vi "Load Application Config.vi"(8 "error in":errorcluster, 10 "Config path":path=path "C:/GitHub/OOP_Submodule EOL/Config/INI Config.ini", 11 "Sequence Context In":refnum<k7>) -> (0 "error out":errorcluster)   [LabVIEW 2021]
uses:
  <vilib>/Utility/config.llb/Read Key (String).vi
  <vilib>/addons/TestStand/_TSUtility.llb/TestStand - Set Property Value (String).vi
  <vilib>/addons/TestStand/_TSUtility.llb/TestStand - Set Property Value (Number).vi
  <vilib>/Utility/config.llb/NI_LVConfig.lvlib
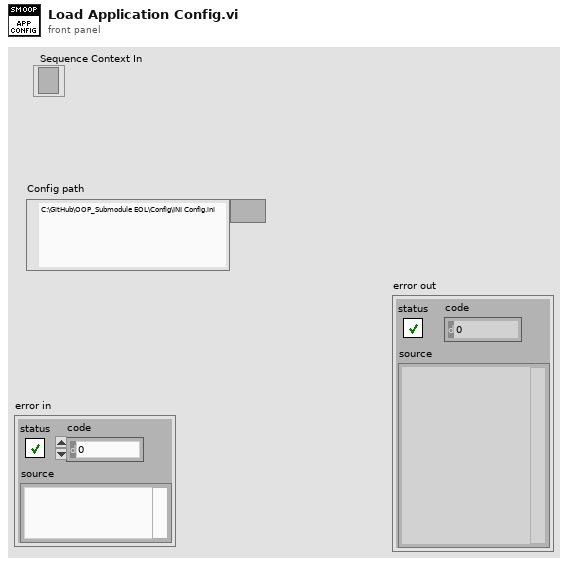
[diagram p1: front panel]
types:
  T1 = typedef "NI_LVConfig.lvlib/Config Data RefNum.ctl" = refnum<k1>
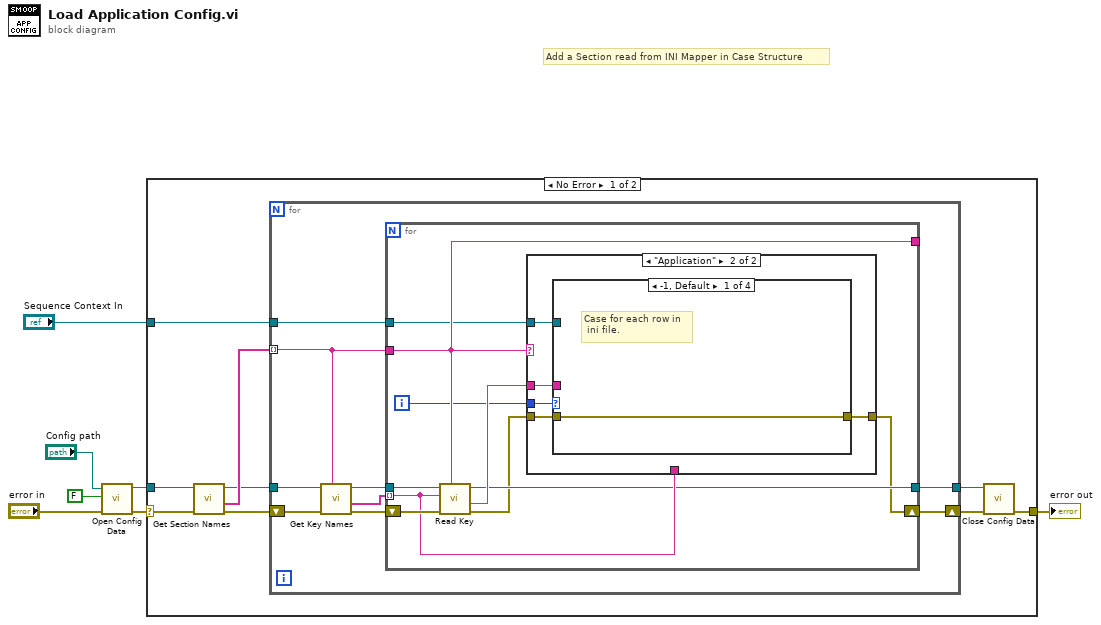
[diagram p0: block diagram]
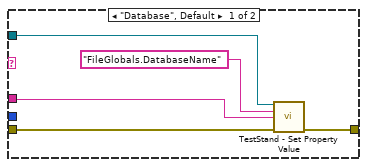
[diagram p2: hidden frame]
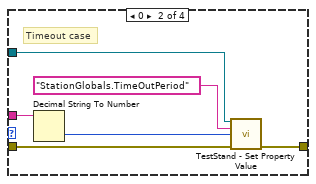
[diagram p3: hidden frame]
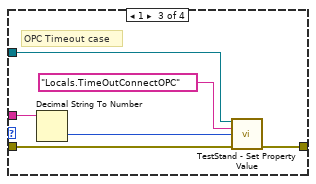
[diagram p4: hidden frame]
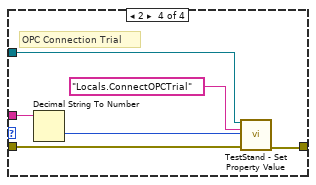
[diagram p5: hidden frame]
diagram:
  # "Add a Section read from INI Mapper in Case Structure"
  n1 = call <vilib>:"Open Config Data.vi"("error in (no error)"="error in", "create file if necessary (T)"=FALSE, "configuration file path"="Config path") -> ("error out"=w5:errorcluster, "refnum"=w6:T1)  [unwired: 6 in, 1 out]
  n2 = case shown="No Error" w5 {
    selector: w5 -> [w16 w65]
    tunnel: [w9 w65] -> w2
    tunnel: w6 -> [w15 _]
    tunnel: "Sequence Context In" -> [w8 _]
    frame No Error {
      n3 = call <vilib>:"Get Section Names.vi"("error in (no error)"=w16, "refnum"=w15) -> ("error out"=w13:errorcluster, "section names"=w14:string[], "refnum out"=w12:T1)  [unwired: 7 in]
      n4 = for {
        tunnel: w14 -> [w22] mode=indexing
        tunnel: w12 -> [w24]
        tunnel: [w23] -> w11
        shift-right: [w18] -> w10
        shift-left: w13 -> [w25]
        tunnel: w8 -> [w17]
        n5 = call <vilib>:"Get Key Names.vi"("section"=w22, "error in (no error)"=w25, "refnum"=w24) -> ("error out"=w21:errorcluster, "key names"=w20:string[], "refnum out"=w19:T1)  [unwired: 5 in, 1 out]
        n6 = for {
          tunnel: w20 -> [w33] mode=indexing
          tunnel: w22 -> [w30]
          tunnel: w19 -> [w34]
          tunnel: [w31] -> w23
          tunnel: [w30] -> _
          shift-right: [w26] -> w18
          shift-left: w21 -> [w35]
          tunnel: w17 -> [w29]
          i -> [w28]
          n7 = call-poly <vilib>:"Read Key.vi"("section"=w30, "error in (no error)"=w35, "key"=w33, "refnum"=w34) -> ("error out"=w27:errorcluster, "value"=w32:string, "refnum out"=w31:T1)  [unwired: 4 in, 1 out]
          n8 = case shown="\"Application\"" w30 {
            tunnel: w33 -> [_ _]
            tunnel: w32 -> [w39 w45]
            tunnel: w29 -> [w38 w43]
            tunnel: w28 -> [_ w44]
            tunnel: w27 -> [w37 w42]
            tunnel: [w36 w41] -> w26
            frame "Database", Default {
              n9 = call-poly <vilib>:"TestStand - Set Property Value.vi"("Sequence Context In"=w38, "Lookup String"="FileGlobals.DatabaseName", "New Value"=w39, "error in (no error)"=w37) -> ("error out"=w36:errorcluster)  [unwired: 10 in, 1 out]
            }
            frame "Application" {
              n10 = case shown="-1, Default" w44 {
                tunnel: w45 -> [_ w51 w57 w63]
                tunnel: w43 -> [_ w49 w55 w61]
                tunnel: w42 -> [w46 w48 w54 w60]
                tunnel: [w46 w47 w53 w59] -> w41
                frame -1, Default {
                  # "Case for each row in\n ini file."
                }
                frame 0 {
                  # "Timeout case"
                  n11 = Decimal String To Number(string=w51) -> (number=w50:i32)  [unwired: 2 in, 1 out]
                  n12 = call-poly <vilib>:"TestStand - Set Property Value.vi"("Sequence Context In"=w49, "Lookup String"="StationGlobals.TimeOutPeriod", "New Value"=w50, "error in (no error)"=w48) -> ("error out"=w47:errorcluster)  [unwired: 10 in, 1 out]
                }
                frame 1 {
                  # "OPC Timeout case"
                  n13 = Decimal String To Number(string=w57) -> (number=w56:i32)  [unwired: 2 in, 1 out]
                  n14 = call-poly <vilib>:"TestStand - Set Property Value.vi"("Sequence Context In"=w55, "Lookup String"="Locals.TimeOutConnectOPC", "New Value"=w56, "error in (no error)"=w54) -> ("error out"=w53:errorcluster)  [unwired: 10 in, 1 out]
                }
                frame 2 {
                  # "OPC Connection Trial"
                  n15 = Decimal String To Number(string=w63) -> (number=w62:i32)  [unwired: 2 in, 1 out]
                  n16 = call-poly <vilib>:"TestStand - Set Property Value.vi"("Sequence Context In"=w61, "Lookup String"="Locals.ConnectOPCTrial", "New Value"=w62, "error in (no error)"=w60) -> ("error out"=w59:errorcluster)  [unwired: 10 in, 1 out]
                }
              }
            }
          }
        }
      }
      n17 = call <vilib>:"Close Config Data.vi"("error in (no error)"=w10, "refnum"=w11) -> ("error out"=w9:errorcluster)  [unwired: 8 in, 1 out]
    }
    frame Error {
    }
  }
  "error out" <- w2
